vi "_Create (Protected).vi"(8 "error in (no error)":errorcluster, 11 "MapImp in":refnum<class "MapImp.lvclass">) -> (0 "error out":errorcluster, 3 "MapImp out":refnum<class "MapImp.lvclass">)   [LabVIEW 2013, in "LapDog.Collections.v1.Maps.lvlib" / "MapImp.lvclass"]
uses:
  MapImp.lvclass
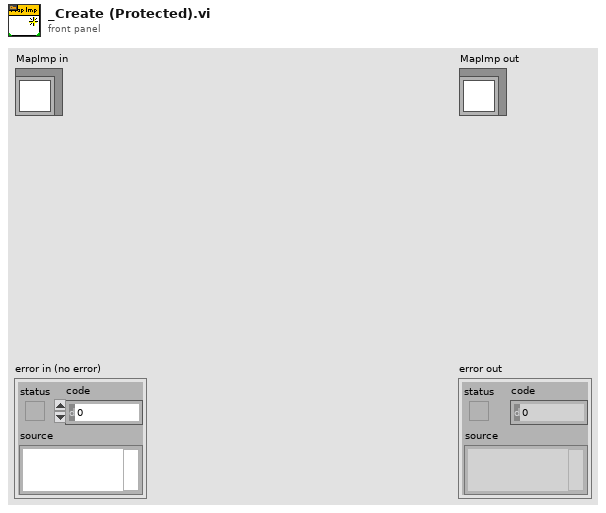
[diagram p1: front panel]
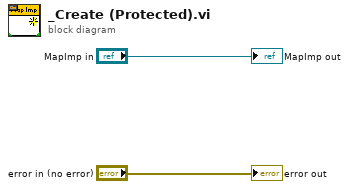
[diagram p0: block diagram]
diagram:
  "error out" <- "error in (no error)"
  "MapImp out" <- "MapImp in"
